vi "L1_ThresholdSweepnWrite.vi"(0 "VISA In":refnum<visa-resource-name>="AgilentOsciloscope", 1 "Channel Register":i32=98, 2 "Vin":dbl=0.3, 3 "File path In":path=path "C:/Users/omartinez/Desktop/L0nL1_Results/L1_SN__DT_Test.csv", 5 "ID In":refnum<k5>, 7 "Error In":errorcluster, 11 "CH":i32, 12 "Active Adder":i32=98, 13 "Digital Output":i32) -> (4 "VISA Out":refnum<visa-resource-name>="AgilentOsciloscope", 6 "ID out":refnum<k5>, 8 "Error Out":errorcluster)   [LabVIEW 2012]
uses:
  Sum_Abrilader/L0_Sum_Adder Folder/C/Program Files/National Instruments/LabVIEW 2012/instr.lib/Agilent 8000 Series/Public/Data/Low Level/Fetch Measurement (More).vi
  <vilib>/Utility/file.llb/Write To Spreadsheet File (DBL).vi
  <instrlib>/Agilent 8000 Series/Agilent 8000 Series.lvlib
panel:
  out "Current DAC value":i32
  out "IPR_count":u32=1000
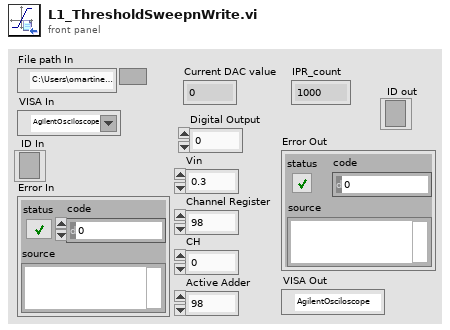
[diagram p1: front panel]
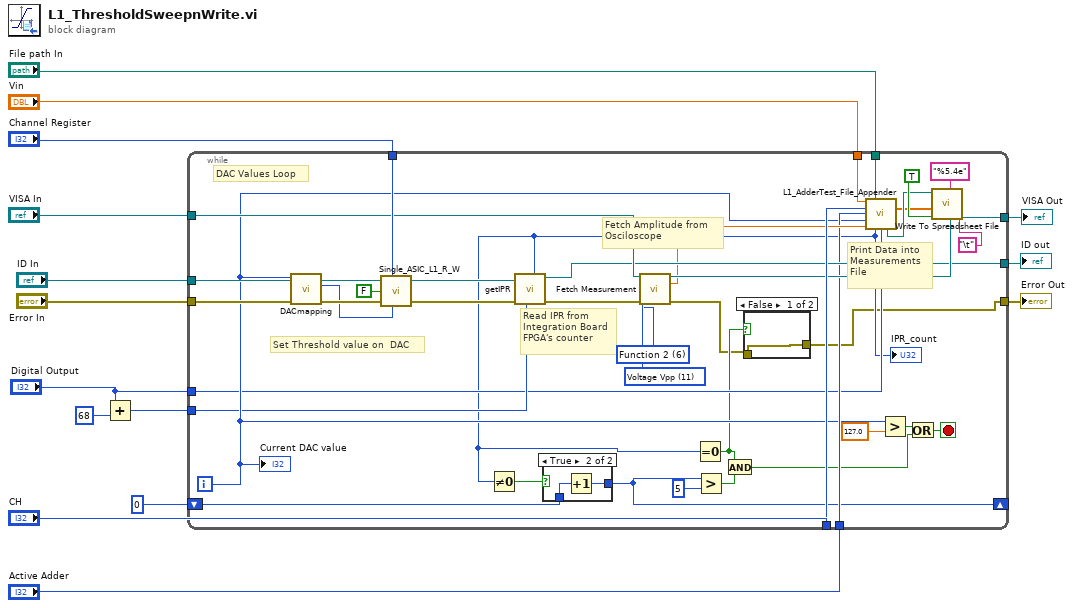
[diagram p0: block diagram]
diagram:
  n1 = Add(x="Digital Output", y=68) -> (x+y=w3:i32)
  n2 = while {
    tunnel: "ID In" -> [w55]
    tunnel: "Channel Register" -> [w53]
    tunnel: "Error In" -> [w52]
    tunnel: [w39] -> w11
    tunnel: [w16] -> w12
    tunnel: "File path In" -> [w49]
    tunnel: "CH" -> [w48]
    tunnel: "Active Adder" -> [w37]
    tunnel: "Vin" -> [w47]
    tunnel: "VISA In" -> [w44]
    tunnel: [w43] -> w10
    tunnel: w3 -> [w34]
    tunnel: "Digital Output" -> [w33]
    shift-right: [w18] -> _
    shift-left: 0 -> [w30]
    i -> [w35]
    stop <- w29 stop-if-true
    w46 = 11 items=["Rise Time", "Fall Time", "Frequency", "Period", "Voltage RMS(AC)", "Voltage RMS(DC)", "Voltage RMS (AC,cycle)", "Voltage RMS (DC,cycle)", "Voltage Max", "Voltage Min", "Voltage Middle", "Voltage Vpp", "Voltage High", "Voltage Low", "Voltage Average", "Voltage Average (cycle)", "Width Negative", "Width Positive", "Duty Cycle Positive", "Amplitude", "Overshoot", "Preshoot", "Voltage Base", "Voltage Upper", "Time Max", "Time Min", "Color Grade Crossing", "Color Grade Eye Width", "Color Grade Eye Height", "Color Grade Eye Q-Factory", "Color Grade Eye Duty Cycle Distortion(Percent)", "Color Grade Eye Duty Cycle Distortion(Time)", "Color Grade Eye Jitter(PP)", "Color Grade Eye Width(RMS)", "Cycle-cycle Duty Jitter(Rising)", "Cycle-cycle Duty Jitter(Falling)", "Cycle-cycle Jitter(Rising)", "Cycle-cycle Jitter(Falling)", "Cycle-cycle - Width", "Cycle-cycle + Width", "Date Rate", "Unit Interval", "FFT Delta Frequency", "FFT Delta Magnitude", "FFT Frequency", "FFT Magnitude", "Slew Rate", "Area (Entire Display)", "Area(Single Cycle)", "Duty Cycle (Rising)", "Duty Cycle (Falling)"] ("Measurement Function (0: Rise Time)")
    w45 = 6 items=["Channel 1"=1, "Channel 2"=2, "Channel 3"=3, "Channel 4"=4, "Function 1"=5, "Function 2"=6, "Function 3"=7, "Function 4"=8, "Memory 1"=9, "Memory 2"=10, "Memory 3"=11, "Memory 4"=12] ("Channel (1: Channel 1)")
    # "Print Data into\nMeasurements \nFile"
    # "Fetch Amplitude from\nOsciloscope"
    # "Read IPR from \nIntegration Board\nFPGA's counter"
    # "Set Threshold value on  DAC"
    # "DAC Values Loop"
    n3 = call "DACmapping.vi"("error in (no error)"=w52, "DAC_TH"=w35) -> ("error out"=w51:errorcluster, "COMB DEC"=w50:u32)  [unwired: 8 in]
    n4 = call "Single_ASIC_L1_R_W.vi"("connection ID"=w55, "Register or channel"=w53, "RD/#WR"=FALSE, "error in (no error)"=w51, "Data"=w50) -> ("connection ID out"=w40:refnum<k5>, "error out"=w42:errorcluster)  [unwired: 1 in, 2 out]
    n5 = call "getIPR.vi"("Address"=w34, "error in"=w42, "connection ID"=w40) -> ("error out"=w41:errorcluster, "connection ID out"=w39:refnum<k5>, "IPR_count"=w20:u32)  [unwired: 5 in, 1 out]
    "IPR_count" <- w20
    n6 = Not Equal To 0?(x=w20) -> (x != 0?=w31:bool)
    n7 = case shown="True" w31 {
      tunnel: w30 -> [w58 w60]
      tunnel: [w58 w59] -> w18
      frame False {
      }
      frame True {
        n8 = Increment(x=w60) -> (x+1=w59:i32)
      }
    }
    n9 = call-poly "Fetch Measurement.vi"("VISA resource name"=w44, "Channel (1: Channel 1)"=w45, "Measurement Function (0: Rise Time)"=w46, "error in (no error)"=w41) -> ("VISA resource name out"=w43:refnum<visa-resource-name>, "Measurement"=w38:dbl, "error out"=w17:errorcluster)  [unwired: 9 in]
    n10 = Equal To 0?(x=w20) -> (x = 0?=w19:bool)
    n11 = Greater?(x=w18, y=5) -> (0:w28:bool)
    n12 = And(x=w19, y=w28) -> (x .and. y?=w27:bool)
    n13 = case shown="False" w19 {
      tunnel: w17 -> [w56 w57]
      tunnel: [w56 w57] -> w16
      frame False {
      }
      frame True {
      }
    }
    n14 = call "L1_AdderTest_File_Appender.vi"("Vin"=w47, "file path (dialog if empty)"=w49, "CH"=w48, "Active Adder"=w37, "DAC Level"=w35, "Vmeas"=w38, "IPR"=w20, "Digital Output"=w33) -> ("appended array"=w24:dbl[], "file path (dialog if empty) 2"=w25:path)  [unwired: 6 in]
    n15 = Greater?(x=w35, y=sgl 127.0) -> (0:w32:bool)
    n16 = Or(x=w32, y=w27) -> (x .or. y?=w29:bool)
    n17 = call-poly <vilib>:"Write To Spreadsheet File.vi"("delimiter (\\t)"="\t", "format (%.;%.3f)"="%5.4e" ("format (%.3f)"), "append to file? (new file:F)"=TRUE, "1D data"=w24, "file path (dialog if empty)"=w25) -> ()  [unwired: 3 in, 1 out]
    "Current DAC value" <- w35
  }
  "Error Out" <- w12
  "ID out" <- w11
  "VISA Out" <- w10
